vi "Get Events.vi"(11 "Project View in":refnum<class "Project View.lvclass">) -> (2 "Events":T1, 3 "Project View out":refnum<class "Project View.lvclass">)   [LabVIEW 2013, in "Project View.lvlib" / "Project View.lvclass"]
uses:
  Project View.lvclass
  Typedef/Events.ctl
  Project View.lvclass/Project View.ctl
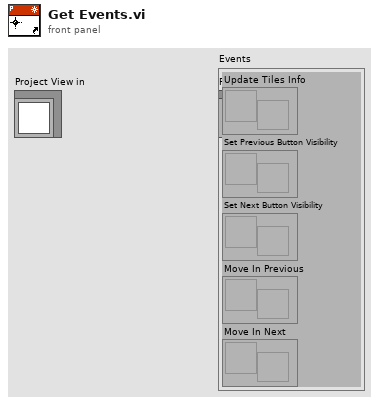
[diagram p1: front panel]
types:
  T1 = typedef "Project View.lvlib/Project View.lvclass/Events.ctl" = cluster{"Update Tiles Info":refnum<user-event>, "Set Previous Button Visibility":refnum<user-event>, "Set Next Button Visibility":refnum<user-event>, "Move In Previous":refnum<user-event>, "Move In Next":refnum<user-event>}
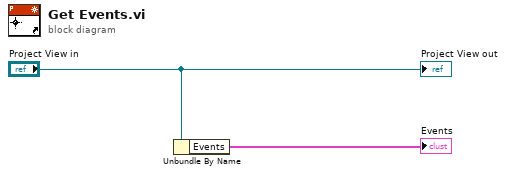
[diagram p0: block diagram]
diagram:
  n1 = Unbundle By Name("Project View in") -> ("Events"=→"Events":T1)
  "Project View out" <- "Project View in"
